vi "testGetEventTask.vi"(8 "error in (no error)":errorcluster) -> (0 "error out":errorcluster)   [LabVIEW 2018]
doc: "Test the task to get the event by LabVIEW. The command line should provide three arguments: (1) path to the SAL LabVIEW monitor, (2) path to the LV Lib, and (3) path of sending event cpp file (summary state)."
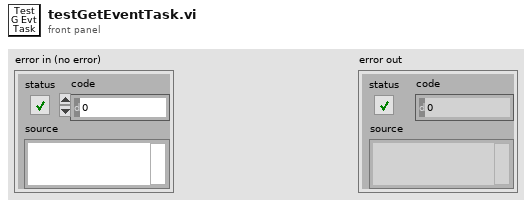
[diagram p1: front panel]
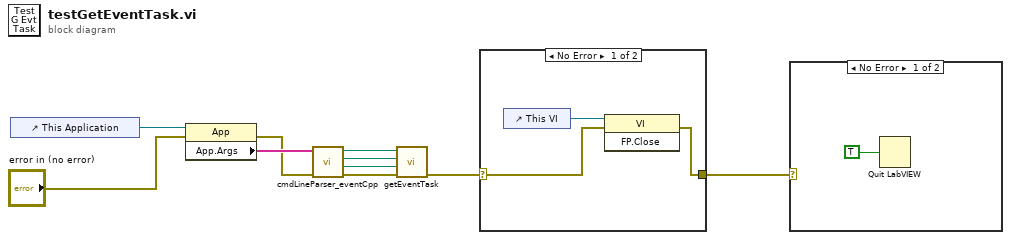
[diagram p0: block diagram]
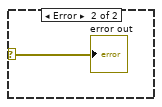
[diagram p2: hidden frame]
diagram:
  n1 = control-ref of="This Application"() -> (w10:refnum<vi>)
  n2 = property class="App"(reference=w10, error in="error in (no error)") -> (error out=w5:errorcluster, "App.Args"=w6:string[])  [unwired: 1 out]
  n3 = call "cmdLineParser_eventCpp.vi"("error in (no error)"=w5, "cmdLineArgs"=w6) -> ("error out"=w4:errorcluster, "pathEventCpp"=w1:path, "pathLvLib"=w2:path, "pathMonitor"=w3:path)  [unwired: 5 in, 1 out]
  n4 = call "getEventTask.vi"("error in (no error)"=w4, "pathOfSendEventSummaryState"=w1, "pathLvLib"=w2, "pathMonitor"=w3) -> ("error out"=w7:errorcluster)  [unwired: 7 in]
  n5 = case shown="No Error" w7 {
    selector: w7 -> [w11 w14]
    tunnel: [w12 w14] -> w8
    frame No Error {
      n6 = control-ref of="This VI"() -> (w13:refnum<vi>)
      n7 = invoke class="VI" method="FP.Close"(reference=w13, error in=w11) -> (error out=w12:errorcluster)  [unwired: 1 in, 2 out]
    }
    frame Error {
    }
  }
  n8 = case shown="No Error" w8 {
    selector: w8 -> [_ w16]
    frame No Error {
      n9 = Quit LabVIEW(quit? (T)=TRUE) -> ()
    }
    frame Error {
      "error out" <- w16
    }
  }
